vi "Append Report Text (num).vi"(0 "report in":refnum<class "NI_HTML.lvclass">, 1 "MS Office parameters":T1, 2 "format string (%.3f)":string="%.3f", 7 "text":dbl format="%.2f", 9 "append on new line? (F)":bool, 11 "error in (no error)":errorcluster) -> (4 "report out":refnum<class "NI_HTML.lvclass">, 8 "start out (Word)":i32, 10 "end out (Word)":i32, 15 "error out":errorcluster)   [LabVIEW 2020, in "NI_HTML.lvclass"]
doc: "Appends text to the selected report."
uses:
  NI_HTML.lvclass
  NI_HTML.lvclass/NI_HTML.ctl
  NI_ReportGenerationCore.lvlib
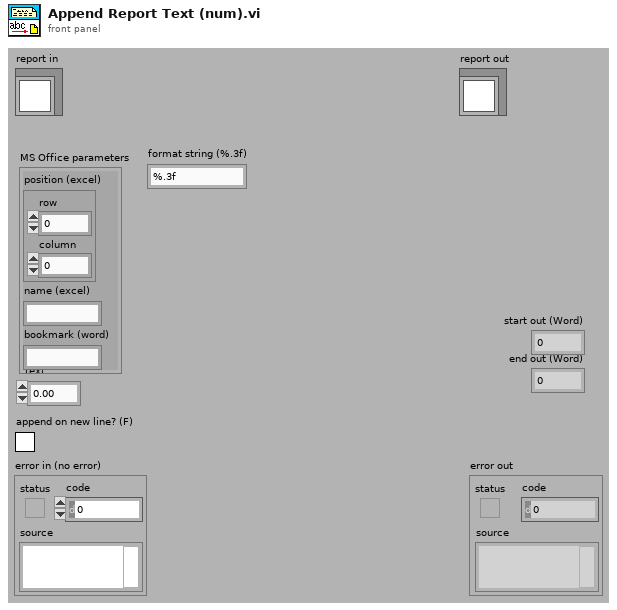
[diagram p1: front panel]
types:
  T1 = cluster{"position (excel)":cluster{"row":i32, "column":i32}, "name (excel)":string, "bookmark (word)":string}
  T2 = typedef "NI_ReportGenerationCore.lvlib/HTML Report Data.ctl" = cluster{"Body Text":string, "Font Tag":string, "Title Text":string, "Header Text":string, "Footer Text":string, "Image List":path[]}
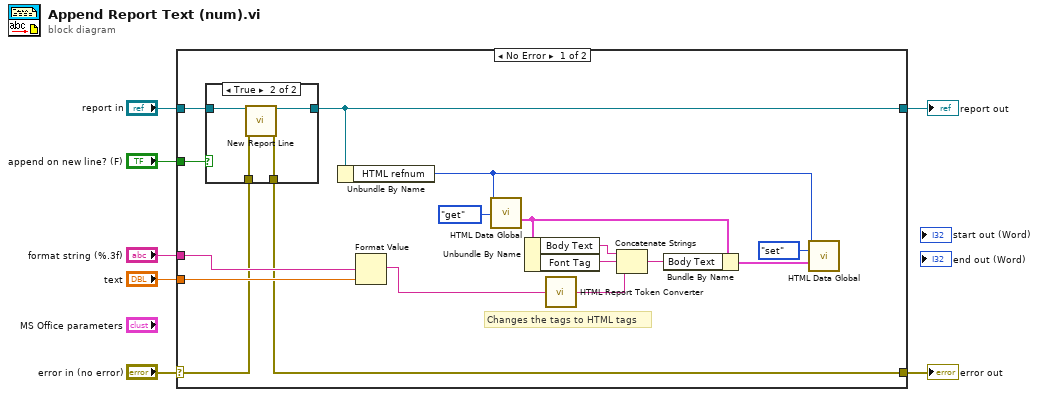
[diagram p0: block diagram]
diagram:
  n1 = case shown="No Error" "error in (no error)" {
    selector: "error in (no error)" -> [w16 w32]
    tunnel: [w15 w32] -> w6
    tunnel: [w13 w31] -> w4
    tunnel: "report in" -> [w24 w31]
    tunnel: "append on new line? (F)" -> [w23 _]
    tunnel: "text" -> [w18 _]
    tunnel: "format string (%.3f)" -> [w17 _]
    frame No Error {
      # "Changes the tags to HTML tags"
      n2 = case shown="True" w23 {
        tunnel: w24 -> [w26 w30]
        tunnel: [w26 w29] -> w13
        tunnel: w16 -> [w25 w28]
        tunnel: [w25 w27] -> w15
        frame False {
        }
        frame True {
          n3 = call-dynamic "New Report Line.vi"("report in"=w30, "error in (no error)"=w28) -> ("report out"=w29:refnum<class "NI_HTML.lvclass">, "error out"=w27:errorcluster)  [unwired: 1 in, 11 out]
        }
      }
      n4 = Unbundle By Name(w13) -> ("HTML refnum"=w8:u32)
      n5 = Format Value(format string=w17, value (0)=w18) -> (output string=w19:string)  [unwired: 1 out]
      n6 = call "HTML Data Global.vi"("HTML refnum"=w8, "menu"=enum16{"init", "get", "set", "delete"}."get") -> ("HTML report data out"=w9:T2)  [unwired: 1 in, 12 out]
      n7 = Unbundle By Name(w9) -> ("Body Text"=w22:string, "Font Tag"=w21:string)
      n8 = call "HTML Report Token Converter.vi"("String In"=w19) -> ("String Out"=w20:string)
      n9 = Concatenate Strings(w22, w21, w20) -> (w10:string)
      n10 = Bundle By Name(cluster=w9, "Body Text"=w10) -> (w11:T2)
      n11 = call "HTML Data Global.vi"("HTML refnum"=w8, "menu"=enum16{"init", "get", "set", "delete"}."set", "HTML report data in"=w11) -> ()  [unwired: 13 out]
    }
    frame Error {
    }
  }
  "error out" <- w6
  "report out" <- w4
